vi "Set_Cluster_Argument0.vi"(1 "Clust Refnum":refnum<vi>, 2 "Argument List In":string[](array[string])) -> (0 "Argument List Out":string[](array[string]))   [LabVIEW 2011]
doc: "This VI parses an argument to find it's text value. For example, given an argument in the form of Arg(\"some text\"), it would return \"some text\", without quotation marks."
uses:
  high_level_proc/source_dilution.ctl
  high_level_proc/source_noDilution.ctl
panel:
  out "error out":errorcluster
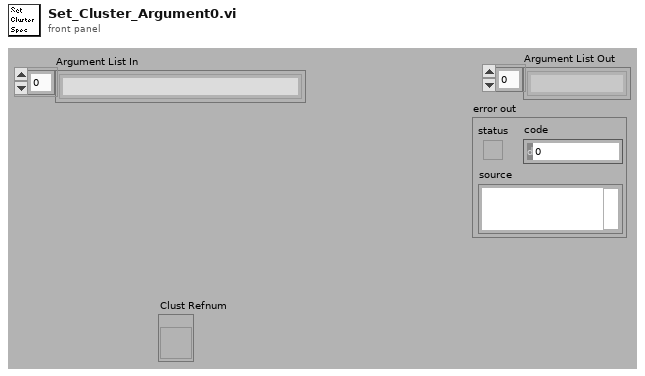
[diagram p1: front panel]
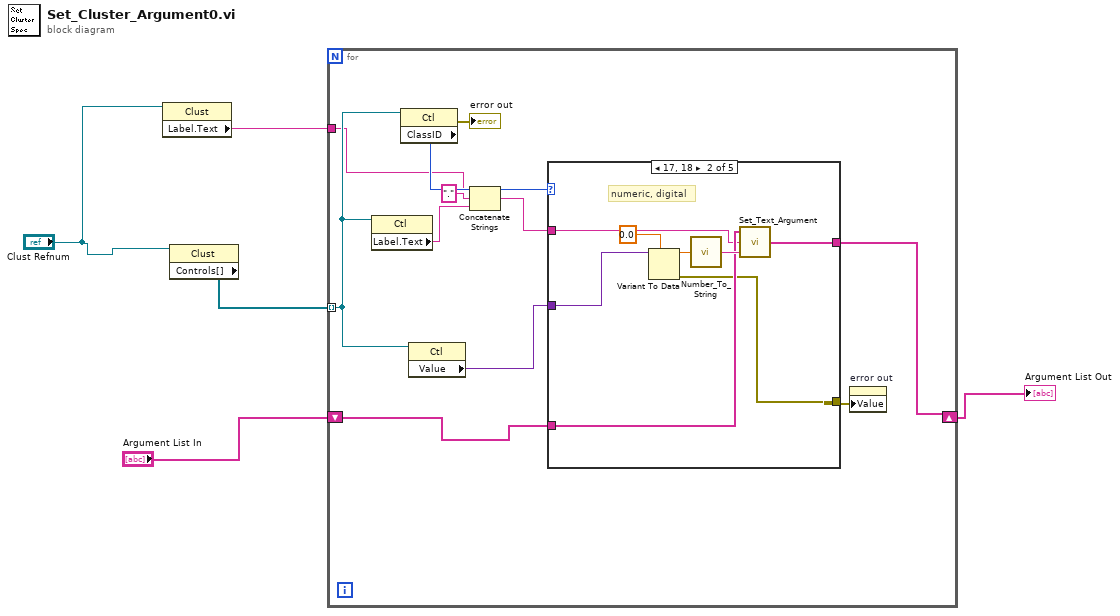
[diagram p0: block diagram]
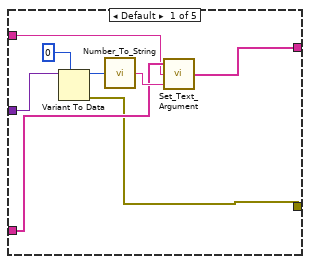
[diagram p2: hidden frame]
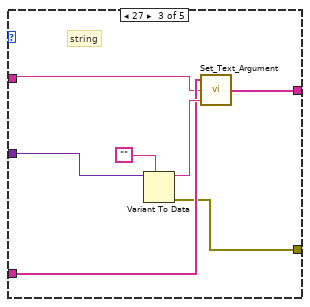
[diagram p3: hidden frame]
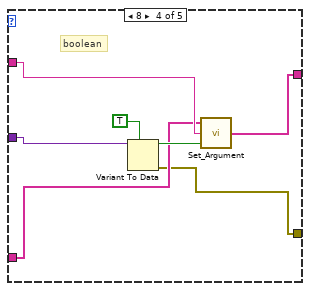
[diagram p4: hidden frame]
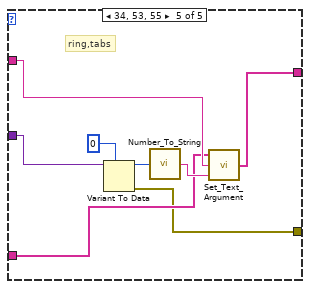
[diagram p5: hidden frame]
diagram:
  n1 = property class="Clust"(reference="Clust Refnum") -> ("Label.Text"=w1:string)  [unwired: 1 in, 2 out]
  n2 = property class="Clust"(reference="Clust Refnum") -> ("Controls[]"=w3:refnum<vi>[])  [unwired: 1 in, 2 out]
  n3 = for {
    tunnel: w3 -> [w16] mode=indexing
    shift-right: [w13] -> w4
    shift-left: "Argument List In" -> [w14]
    tunnel: w1 -> [w6]
    n4 = property class="Ctl"(reference=w16) -> ("Label.Text"=w9:string)  [unwired: 1 in, 2 out]
    n5 = property class="Ctl"(reference=w16) -> (error out=→"error out":errorcluster, "ClassID"=w15:u32)  [unwired: 1 in, 1 out]
    n6 = property class="Ctl"(reference=w16) -> ("Value"=w12:variant)  [unwired: 1 in, 2 out]
    n7 = Concatenate Strings(w6, "." ("string"), w9) -> (w7:string)
    n8 = case shown="17, 18" w15 {
      tunnel: w14 -> [w21 w29 w37 w43 w49]
      tunnel: [w17 w28 w34 w41 w47] -> w13
      tunnel: w7 -> [w20 w27 w36 w44 w50]
      tunnel: w12 -> [w19 w26 w33 w40 w51]
      tunnel: [w18 w25 w35 w42 w48] -> w10
      frame Default {
        n9 = Variant To Data(type=0, Variant=w19) -> (data=w22:i32, error out=w18:errorcluster)  [unwired: 1 in]
        n10 = call "Number_To_String.vi"("Number"=w22) -> ("String"=w24:string)
        n11 = call "Set_Text_Argument.vi"("Text"=w24, "Argument"=w20, "Argument List In"=w21) -> ("Argument List Out"=w17:string[])
      }
      frame 17, 18 {
        # "numeric, digital"
        n12 = Variant To Data(type=0.0, Variant=w26) -> (data=w31:dbl, error out=w25:errorcluster)  [unwired: 1 in]
        n13 = call "Number_To_String.vi"("Number"=w31) -> ("String"=w30:string)
        n14 = call "Set_Text_Argument.vi"("Text"=w30, "Argument"=w27, "Argument List In"=w29) -> ("Argument List Out"=w28:string[])
      }
      frame 27 {
        # "string"
        n15 = Variant To Data(type="", Variant=w33) -> (data=w38:string, error out=w35:errorcluster)  [unwired: 1 in]
        n16 = call "Set_Text_Argument.vi"("Text"=w38, "Argument"=w36, "Argument List In"=w37) -> ("Argument List Out"=w34:string[])
      }
      frame 8 {
        # "boolean"
        n17 = Variant To Data(type=TRUE, Variant=w40) -> (data=w45:bool, error out=w42:errorcluster)  [unwired: 1 in]
        n18 = call "Set_Argument.vi"("Enable"=w45, "Argument"=w44, "Argument List In"=w43) -> ("Argument List Out"=w41:string[])
      }
      frame 34, 53, 55 {
        # "ring,tabs"
        n19 = Variant To Data(type=u16 0, Variant=w51) -> (data=w52:u16, error out=w48:errorcluster)  [unwired: 1 in]
        n20 = call "Number_To_String.vi"("Number"=w52) -> ("String"=w54:string)
        n21 = call "Set_Text_Argument.vi"("Text"=w54, "Argument"=w50, "Argument List In"=w49) -> ("Argument List Out"=w47:string[])
      }
    }
    n22 = property on="error out" class="Clust (strict)"("Value"=w10) -> ()  [unwired: 2 in, 2 out]
  }
  "Argument List Out" <- w4
